vi "test6_auto.vi"() -> ()   [LabVIEW 2014]
uses:
  <vilib>/LabVIEW Targets/FPGA/cRIO/cRIO-9505/controls.llb/_nicrio_cRIO-9505_DriveDirection.ctl
  <vilib>/rvi/Emulation/niFpgaGetClockAttributes.vi
  <vilib>/rvi/Emulation/niFpgaSctlEmulationGetInTimedLoop.vi
  <vilib>/rvi/Emulation/niFpgaEmulationReportErrorSimple.vi
  <vilib>/rvi/Emulation/niFpgaProcessEmulError.vi
  <vilib>/rvi/eio/common/nirviEmuTemplateMethod_errors.vi
  <vilib>/rvi/Emulation/niFpgaCriticalErrorInLSC.vi
  <vilib>/eio/EIOMethodNode/EIOMethodNode.xnode
  <vilib>/eio/EIONode/EIONode.xnode
panel:
  in  "Encoder_stop":bool
  in  "Motor stop":bool
  out "Motor_Tick Count(Ticks)":u32
  in  "duty cycle (periods)":fxp<+,32,0>
  in  "Mod1/Drive Direction":T1=enum."Counterclockwise"
  out "Mod1/Current Sense":i16
  in  "Mod1/Motor":bool
  out "Encoder_Tick Count(uSec)":u32 caption="Encoder_Tick Count(Ticks)"
  out "Mod1/Encoder Phase A":bool
  out "Mod1/Encoder Phase B":bool
  in  "Position Reset":bool
  in  "Velocity Interval (uSec)":u32=500000
  out "Position (Degrees)":sgl
  out "Acceleration (Counts/Interval)":i32
  out "Velocity (Degrees/Second)":sgl
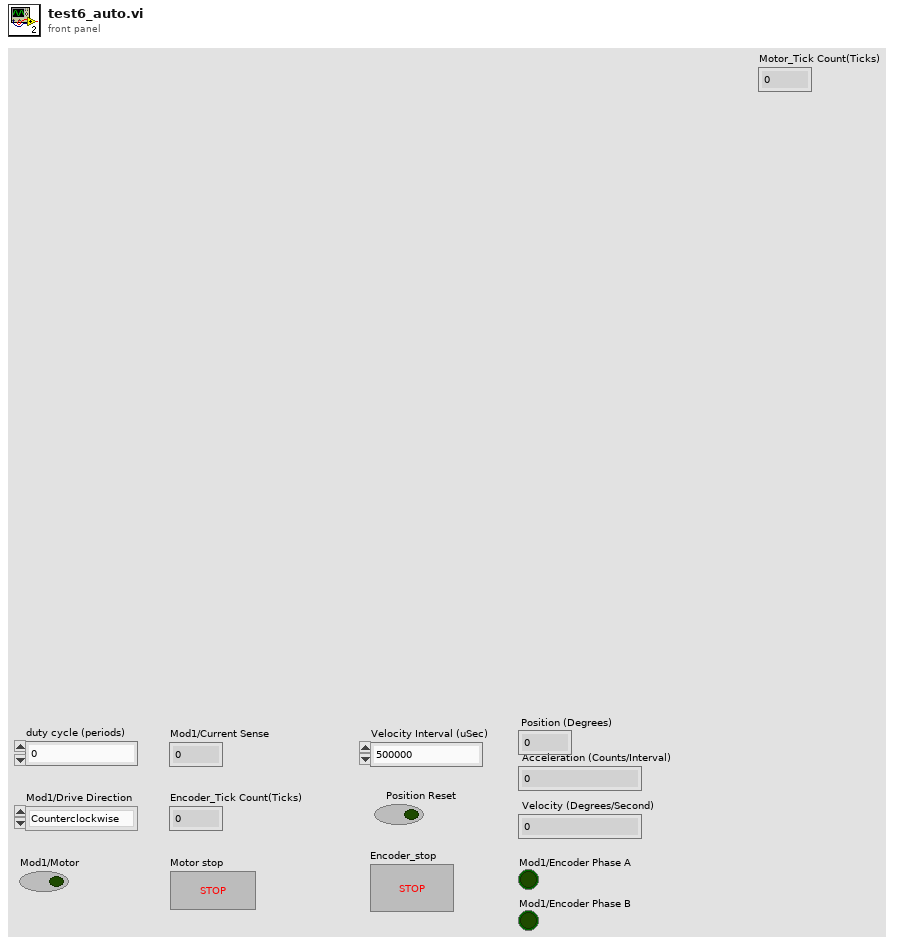
[diagram p1: front panel]
types:
  T1 = typedef "_nicrio_cRIO-9505_DriveDirection.ctl" = enum8{"Clockwise", "Counterclockwise"}
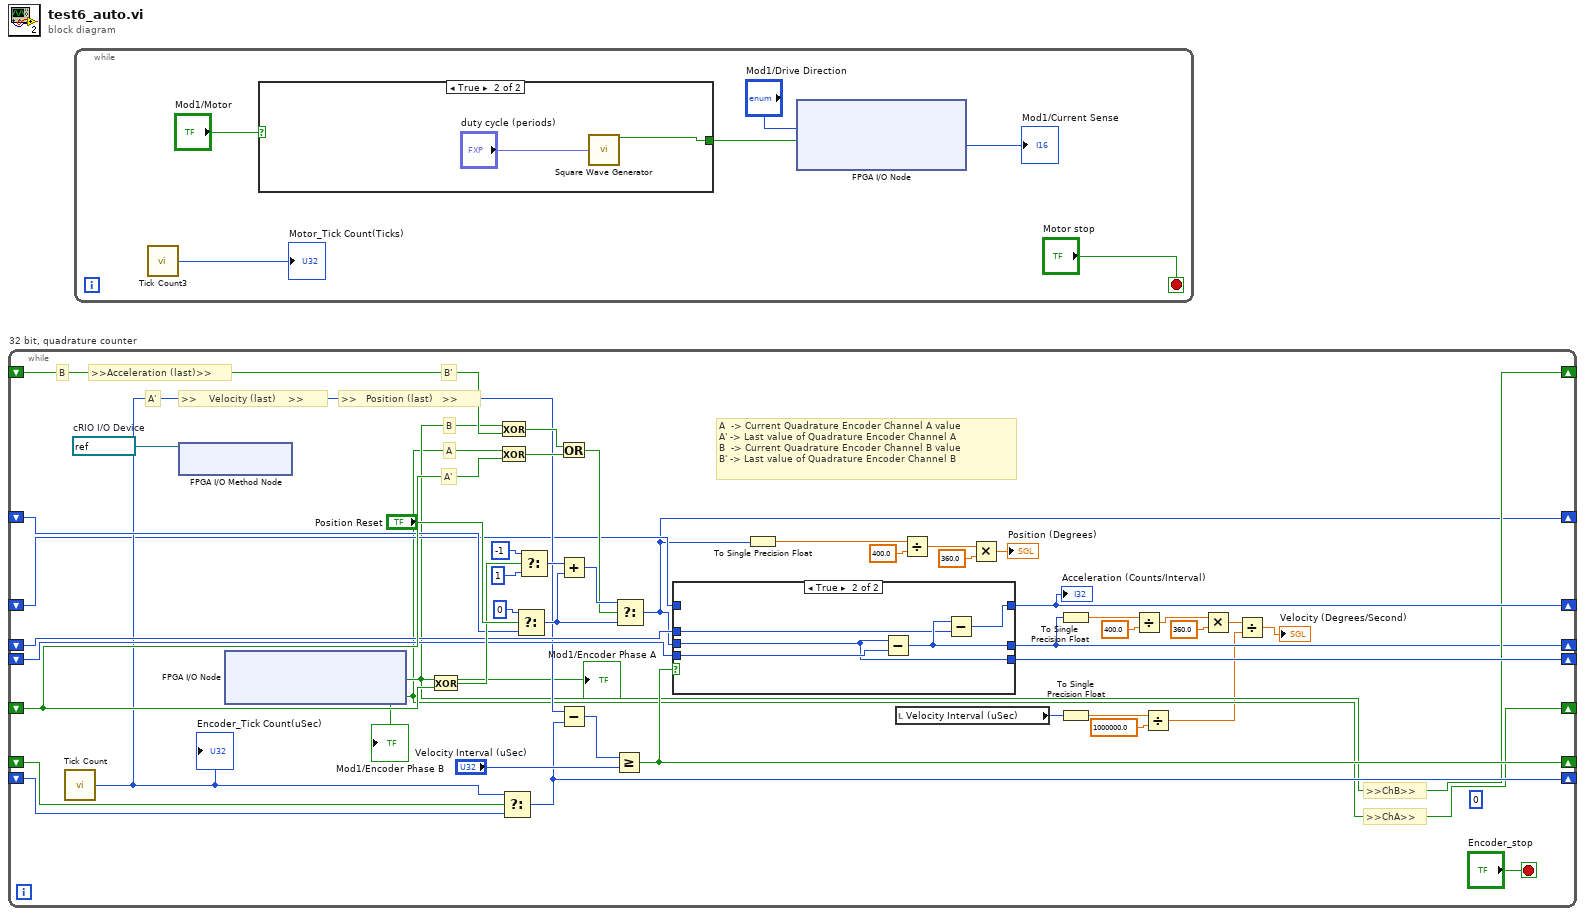
[diagram p0: block diagram]
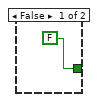
[diagram p2: hidden frame]
diagram:
  n1 = while "32 bit, quadrature counter" {
    shift-right: [w21] -> _
    shift-left: _ -> [w24]
    shift-right: [w17] -> _
    shift-left: _ -> [w35]
    shift-right: [w20] -> _
    shift-left: _ -> [w37]
    shift-right: [w31] -> _
    shift-left: _ -> [w34]
    shift-right: [w26] -> _
    shift-left: _ -> [w32]
    shift-right: [w22] -> _
    shift-left: _ -> [w29]
    shift-right: [w9] -> _
    shift-left: _ -> [w28]
    shift-right: [w23] -> _
    shift-left: _ -> [w25]
    stop <- "Encoder_stop" stop-if-true
    (unwired) i16 0
    w19 = refnum<k21> "Mod1"  # cRIO I/O Device
    # "A  -> Current Quadrature Encoder Channel A value\nA' -> Last value of Quadrature Encoder Channel A\nB  -> Current Quadrature Encoder Channel B value\nB' -> Last value of Quadrature Encoder Channel B"
    # ">>Acceleration (last)>>"
    # "A'"
    # "B"
    # "A'"
    # "A"
    # "B'"
    # "B"
    # ">>ChB>>"
    # ">>ChA>>"
    # ">>    Velocity (last)    >>"
    # ">>   Position (last)   >>"
    n2 = call "Tick Count"() -> ("Tick Count(uSec)"=w27:u32)
    "Encoder_Tick Count(uSec)" <- w27
    n3 = xnode "FPGA I/O Method Node"("FPGA I/O In"=w19) -> ()  [unwired: 1 out]
    n4 = xnode "FPGA I/O Node"() -> ("Mod1/Encoder Phase A"=w21:bool, "Mod1/Encoder Phase B"=w20:bool)  [unwired: 2 in, 2 out]
    "Mod1/Encoder Phase B" <- w20
    "Mod1/Encoder Phase A" <- w21
    n5 = Exclusive Or(1:w37, 2:w21) -> (0:w38:bool)
    n6 = Exclusive Or(1:w24, 2:w21) -> (0:w39:bool)
    n7 = Exclusive Or(1:w37, 2:w20) -> (0:w40:bool)
    n8 = Select(t=w27, s=w34, f=w32) -> (s? t:f=w26:u32)
    n9 = Select(t=0 ("32 bit"), s="Position Reset", f=w35) -> (s? t:f=w45:i32)
    n10 = Select(t=-1 ("32 bit"), s=w38, f=1 ("32 bit")) -> (s? t:f=w43:i32)
    n11 = Or(x=w39, y=w40) -> (x .or. y?=w36:bool)
    n12 = Add(x=w43, y=w45) -> (x+y=w47:i32)
    n13 = Subtract(x=w27, y=w26) -> (x-y=w30:u32)
    n14 = Greater Or Equal?(x=w30, y="Velocity Interval (uSec)") -> (x >= y?=w31:bool)
    n15 = Select(t=w47, s=w36, f=w45) -> (s? t:f=w17:i32)
    n16 = case shown="True" w31 {
      tunnel: w17 -> [_ w51]
      tunnel: w29 -> [w48 w55]
      tunnel: [w50 w54] -> w9
      tunnel: w28 -> [w50 w53]
      tunnel: [w49 w52] -> w23
      tunnel: w25 -> [w49 _]
      tunnel: [w48 w51] -> w22
      frame False {
      }
      frame True {
        n17 = Subtract(x=w51, y=w55) -> (x-y=w54:i32)
        n18 = Subtract(x=w54, y=w53) -> (x-y=w52:i32)
      }
    }
    "Acceleration (Counts/Interval)" <- w23
    n19 = To Single Precision Float(number=w17) -> (single precision float=w16:sgl)
    n20 = local read "Velocity Interval (uSec)"() -> (w6:u32)
    n21 = Divide(x=w16, y=sgl 400.0) -> (x/y=w15:sgl)
    n22 = Multiply(x=w15, y=sgl 360.0) -> (x*y=→"Position (Degrees)":sgl)
    n23 = To Single Precision Float(number=w9) -> (single precision float=w11:sgl)
    n24 = To Single Precision Float(number=w6) -> (single precision float=w5:sgl)
    n25 = Divide(x=w11, y=sgl 400.0) -> (x/y=w12:sgl)
    n26 = Divide(x=w5, y=sgl 1000000.0) -> (x/y=w3:sgl)
    n27 = Multiply(x=w12, y=sgl 360.0) -> (x*y=w8:sgl)
    n28 = Divide(x=w8, y=w3) -> (x/y=→"Velocity (Degrees/Second)":sgl)
  }
  n29 = while {
    stop <- "Motor stop" stop-if-true
    n30 = call "Tick Count3"() -> ("Tick Count(Ticks)"=→"Motor_Tick Count(Ticks)":u32)
    n31 = case shown="True" "Mod1/Motor" {
      tunnel: [FALSE ("square wave out") w64] -> w60
      frame False {
      }
      frame True {
        n32 = call "Square Wave Generator"("duty cycle (periods)"="duty cycle (periods)") -> ("square wave out"=w64:bool)  [unwired: 14 in]
      }
    }
    n33 = xnode "FPGA I/O Node"("Mod1/Drive Direction"="Mod1/Drive Direction", "Mod1/Motor"=w60) -> ("Mod1/Current Sense"=→"Mod1/Current Sense":i16)  [unwired: 3 in, 3 out]
  }
